vi "Create.vi"(8 "Error In":errorcluster[](array[cluster])) -> (0 "Error Out":errorcluster[](array[cluster]), 3 "Bus out":refnum<class "Bus.lvclass">)   [LabVIEW 2014, in "Bus_class.lvlib" / "Bus.lvclass"]
uses:
  Bus.lvclass
  Framework.lvlib
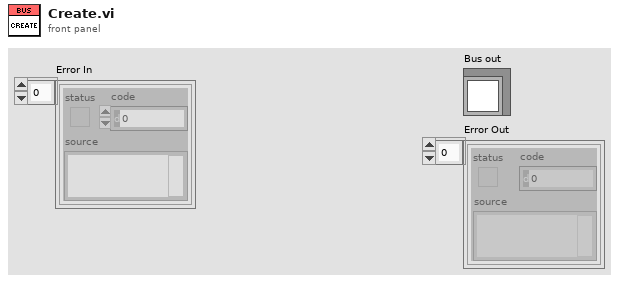
[diagram p1: front panel]
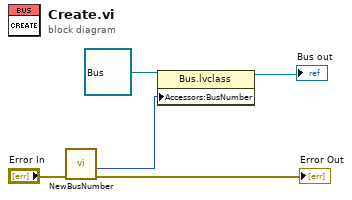
[diagram p0: block diagram]
diagram:
  n1 = call "NewBusNumber.vi"("ErrorArray In"="Error In") -> ("ErrorArray Out"=→"Error Out":errorcluster[], "BusNumber"=w3:u8)  [unwired: 9 in]
  n2 = property class="Bus.lvclass"(reference=refnum<class "Bus.lvclass"> refnum ("Bus_class.lvlib:Bus.lvclass"), "Accessors:BusNumber"=w3) -> (reference out=→"Bus out":refnum<class "Bus.lvclass">)  [unwired: 1 in, 1 out]
